vi "Teleop.vi"(0 "Call Context":T11, 1 "Input":T1) -> (6 "SubState 3":T5, 8 "SubState 4":T5, 9 "SubState 5":T10, 11 "Loop 3 Data":T6, 13 "Loop 4 Data":T4, 14 "SubState 0":T5=enum."driver control", 15 "Loop 1 Data":T8, 16 "Loop 0 Data":T9, 17 "SubState 1":T5, 18 "Loop 2 Data":T7, 19 "SubState 2":T5)   [LabVIEW 2013]
uses:
  typedefs/subStates.ctl
  <vilib>/Rock Robotics/WPI/DriverStation/WPI_DriverStationDerivedRobotMode.ctl
  typedefs/singleUseSubstate.ctl
  typedefs/Loop Datatypes/Loop 0 Datatype.ctl
  typedefs/Loop Datatypes/Loop 1 Datatype.ctl
  typedefs/Loop Datatypes/Loop 2 Datatype.ctl
  typedefs/Loop Datatypes/Loop 3 Datatype.ctl
  typedefs/Loop Datatypes/Loop 4 Datatype.ctl
  <vilib>/Rock Robotics/WPI/Joystick/WPI_JoystickDevRef.ctl
  <vilib>/Rock Robotics/WPI/Joystick/WPI_JoystickDeviceEnum.ctl
  <vilib>/Rock Robotics/WPI/Joystick/WPI_JoystickGetSetRefNum.vi
panel:
  out "JS Axis 2":dbl
  out "JS Axis 1":dbl
  out "JS3":T2
  out "JS1":T2
  out "JS2":T2
  out "Exit Value":i32=-1
  # "Loop Data and Substates"
  # "Latch Loop"
  # "Drive Loop"
  # "Shooter Pneumatics Loop"
  # "Pickup/Passing Belts Loop"
  # "Pickup Arm Loop"
  # "Shifter Loop"
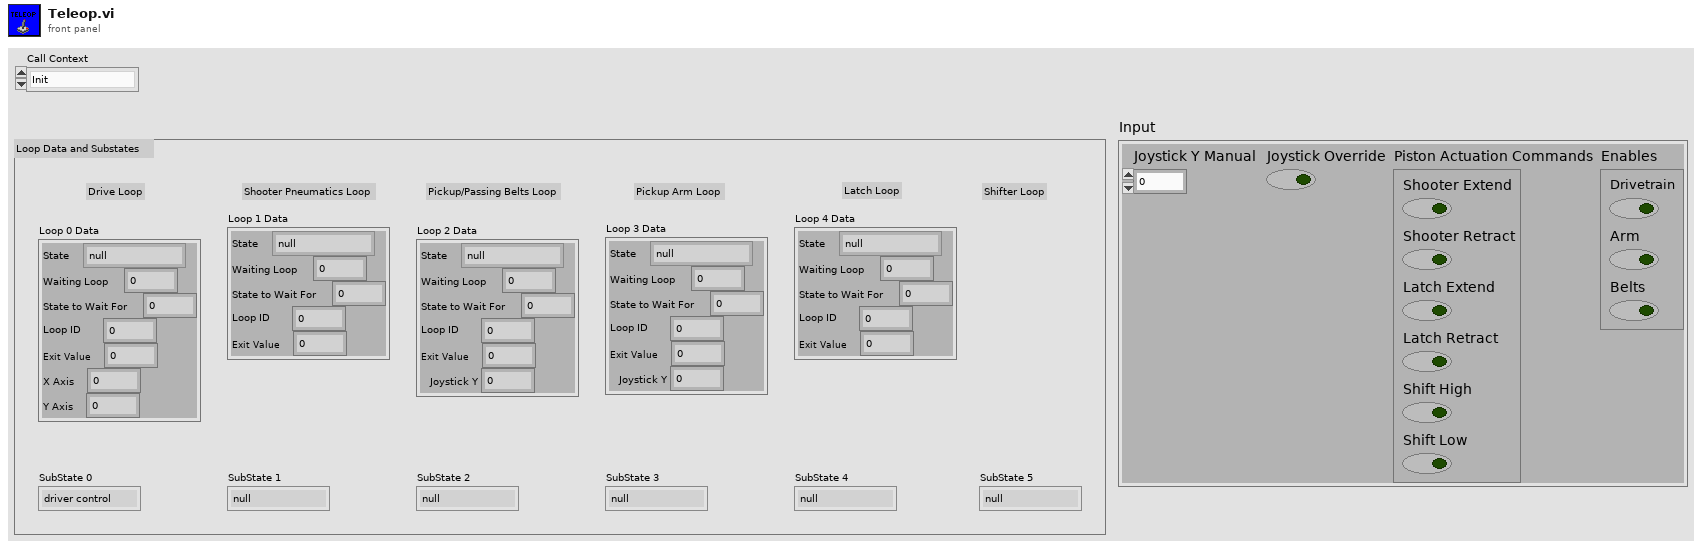
[diagram p1: front panel]
types:
  T1 = cluster{"Joystick Y Manual":dbl, "Joystick Override":bool, "Piston Actuation Commands":cluster{"Shooter Extend":bool, "Shooter Retract":bool, "Latch Extend":bool, "Latch Retract":bool, "Shift High":bool, "Shift Low":bool}, "Enables":cluster{"Drivetrain":bool, "Arm":bool, "Belts":bool}}
  T2 = typedef "WPI_JoystickDevRef.ctl" = cluster{"Device":T3}
  T3 = typedef "WPI_JoystickDeviceEnum.ctl" = enum16{"USB 1", "USB 2", "USB 3", "USB 4", "Kinect 1", "Kinect 2"}
  T4 = typedef "Loop 4 Datatype.ctl" = cluster{"State":T5, "Waiting Loop":i32, "State to Wait For":i32, "Loop ID":i32, "Exit Value":i32}
  T5 = typedef "subStates.ctl" = enum16{"null", "wait", "driver control", "auto", "manual override", "hold position", "rotate", "pickup", "pass", "load", "goto shoot", "shoot", "cancel", "end"}
  T6 = typedef "Loop 3 Datatype.ctl" = cluster{"State":T5, "Waiting Loop":i32, "State to Wait For":i32, "Loop ID":i32, "Exit Value":i32, "Joystick Y":dbl}
  T7 = typedef "Loop 2 Datatype.ctl" = cluster{"State":T5, "Waiting Loop":i32, "State to Wait For":i32, "Loop ID":i32, "Exit Value":i32, "Joystick Y":dbl}
  T8 = typedef "Loop 1 Datatype.ctl" = cluster{"State":T5, "Waiting Loop":i32, "State to Wait For":i32, "Loop ID":i32, "Exit Value":i32}
  T9 = typedef "Loop 0 Datatype.ctl" = cluster{"State":T5, "Waiting Loop":i32, "State to Wait For":i32, "Loop ID":i32, "Exit Value":i32, "X Axis":dbl, "Y Axis":dbl}
  T10 = typedef "singleUseSubstate.ctl" = enum16{"null", "wait", "shift high", "shift low"}
  T11 = typedef "WPI_DriverStationDerivedRobotMode.ctl" = enum16{"Init", "Execute", "Stop"}
  T12 = cluster{"Shooter Extend":bool, "Shooter Retract":bool, "Latch Extend":bool, "Latch Retract":bool, "Shift High":bool, "Shift Low":bool}
  T13 = cluster{"Drivetrain":bool, "Arm":bool, "Belts":bool}
  T14 = cluster{"axis 1 (x)":dbl, "axis 2 (y)":dbl, "axis 3 (throttle)":dbl, "axis 4":dbl, "axis 5":dbl, "axis 6":dbl}
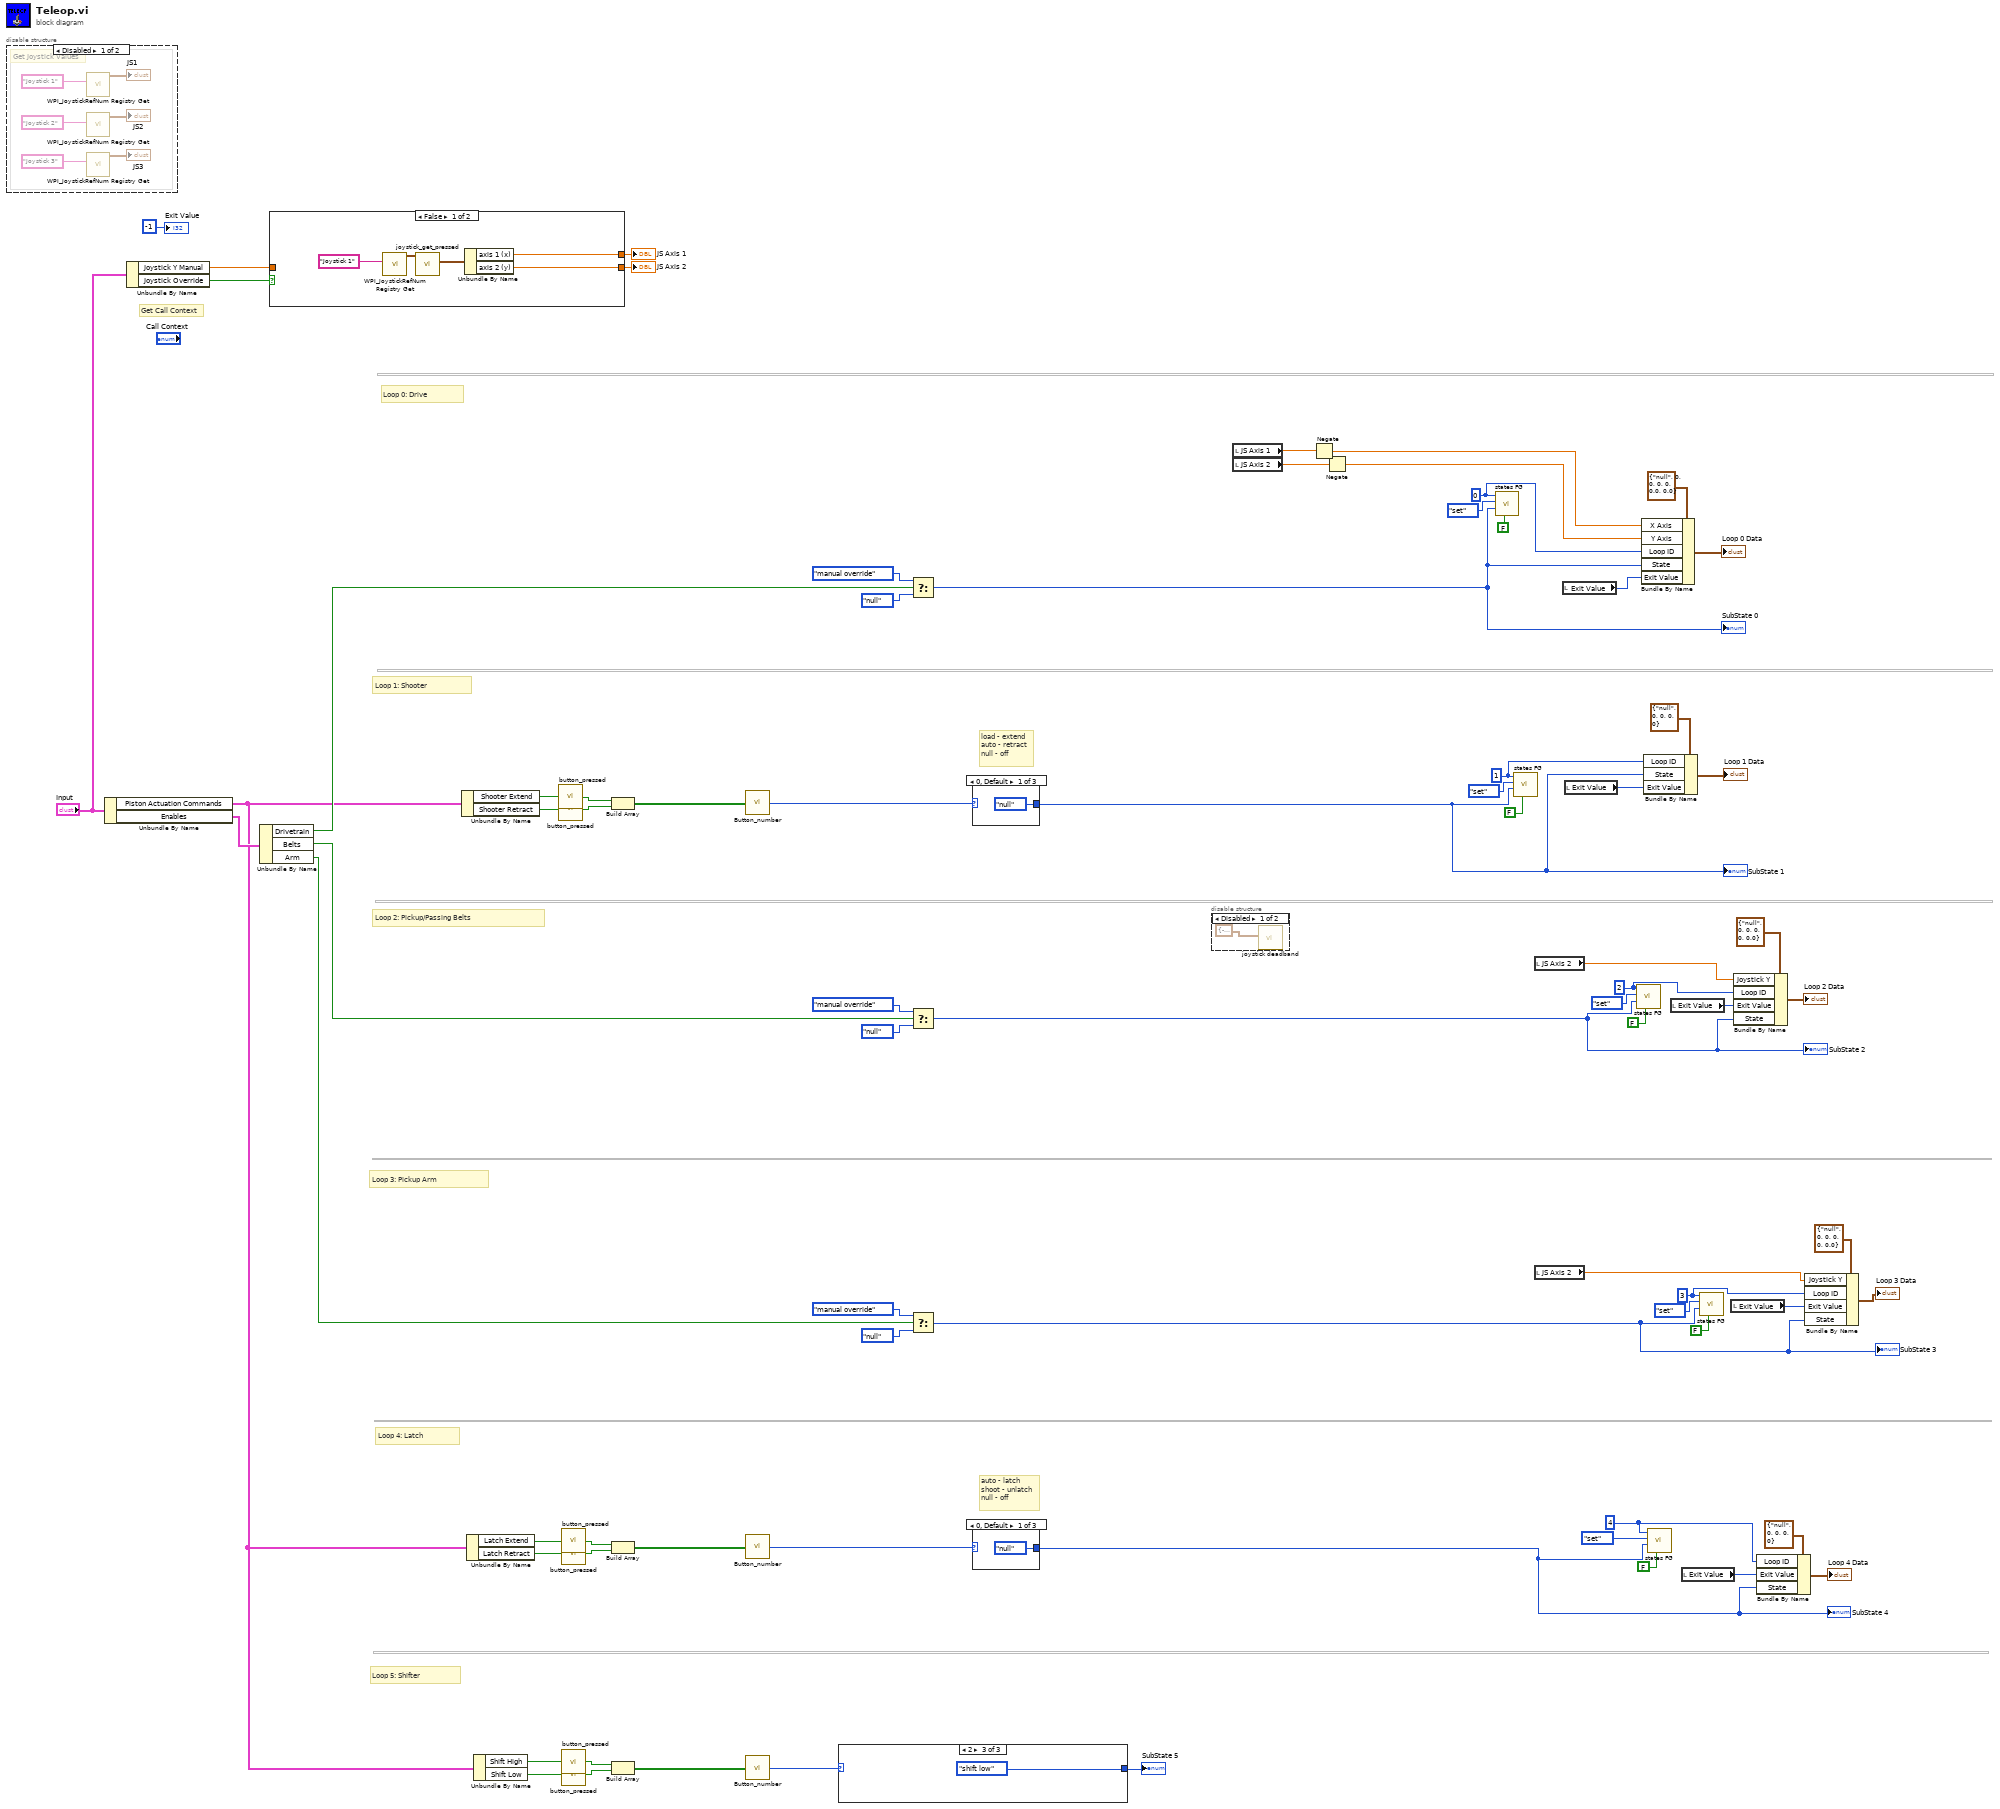
[diagram p0: block diagram]
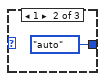
[diagram p5: hidden frame]
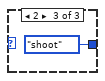
[diagram p6: hidden frame]
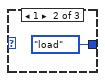
[diagram p7: hidden frame]
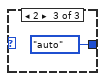
[diagram p8: hidden frame]
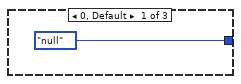
[diagram p9: hidden frame]
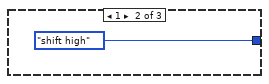
[diagram p10: hidden frame]
diagram:
  w45 = 4 ("Loop ID")
  w58 = 3 ("Loop ID")
  w59 = 2 ("Loop ID")
  w68 = 1 ("Loop ID")
  w70 = 0 ("Loop ID")
  # "auto - latch\nshoot - unlatch\nnull - off"
  # "load - extend\nauto - retract\nnull - off"
  # "Get Call Context"
  # "Loop 4: Latch"
  # "Loop 3: Pickup Arm"
  # "Loop 5: Shifter"
  # "Loop 2: Pickup/Passing Belts"
  # "Loop 1: Shooter"
  # "Loop 0: Drive"
  n1 = disable-structure shown="Disabled" {
    frame Disabled {
      # "Get Joystick Values"
      n2 = call <vilib>:"WPI_JoystickRefNum Registry Get.vi"("refnum name"="Joystick 1") -> ("JoystickDevRef"=→"JS1":T2)  [unwired: 9 in, 1 out]
      n3 = call <vilib>:"WPI_JoystickRefNum Registry Get.vi"("refnum name"="Joystick 2") -> ("JoystickDevRef"=→"JS2":T2)  [unwired: 9 in, 1 out]
      n4 = call <vilib>:"WPI_JoystickRefNum Registry Get.vi"("refnum name"="Joystick 3") -> ("JoystickDevRef"=→"JS3":T2)  [unwired: 9 in, 1 out]
    }
    frame Enabled {
    }
  }
  n5 = Unbundle By Name("Input") -> ("Piston Actuation Commands"=w22:T12, "Enables"=w43:T13)
  n6 = Unbundle By Name("Input") -> ("Joystick Y Manual"=w19:dbl, "Joystick Override"=w20:bool)
  n7 = Unbundle By Name(w43) -> ("Drivetrain"=w42:bool, "Belts"=w36:bool, "Arm"=w31:bool)
  n8 = case shown="False" w20 {
    tunnel: w19 -> [_ w89]
    tunnel: [w84 w89] -> w17
    tunnel: [w85 w89] -> w18
    frame False {
      n9 = call <vilib>:"WPI_JoystickRefNum Registry Get.vi"("refnum name"="Joystick 1") -> ("JoystickDevRef"=w87:T2)  [unwired: 9 in, 1 out]
      n10 = call "joystick_get_pressed.vi"("JoystickDevRef 2"=w87) -> ("Axes"=w86:T14)  [unwired: 1 in, 3 out]
      n11 = Unbundle By Name(w86) -> ("axis 1 (x)"=w85:dbl, "axis 2 (y)"=w84:dbl)
    }
    frame True {
    }
  }
  "JS Axis 1" <- w18
  "JS Axis 2" <- w17
  n12 = Unbundle By Name(w22) -> ("Shooter Extend"=w12:bool, "Shooter Retract"=w10:bool)
  n13 = Unbundle By Name(w22) -> ("Latch Extend"=w7:bool, "Latch Retract"=w8:bool)
  n14 = Unbundle By Name(w22) -> ("Shift High"=w3:bool, "Shift Low"=w4:bool)
  n15 = call "button_pressed.vi"("Button In"=w12) -> ("Button Pressed?"=w11:bool)
  n16 = call "button_pressed.vi"("Button In"=w10) -> ("Button Pressed?"=w9:bool)
  n17 = call "button_pressed.vi"("Button In"=w7) -> ("Button Pressed?"=w6:bool)
  n18 = call "button_pressed.vi"("Button In"=w8) -> ("Button Pressed?"=w5:bool)
  n19 = call "button_pressed.vi"("Button In"=w3) -> ("Button Pressed?"=w2:bool)
  n20 = call "button_pressed.vi"("Button In"=w4) -> ("Button Pressed?"=w1:bool)
  n21 = Build Array(w11, w9) -> (w30:bool[])
  n22 = Build Array(w6, w5) -> (w26:bool[])
  n23 = Build Array(w2, w1) -> (w24:bool[])
  n24 = call "Button_number.vi"("Button Array"=w30) -> ("Button Pressed"=w29:i32)
  n25 = call "Button_number.vi"("Button Array"=w26) -> ("Button Pressed"=w27:i32)
  n26 = call "Button_number.vi"("Button Array"=w24) -> ("Button Pressed"=w23:i32)
  n27 = case shown="2" w23 {
    tunnel: [singleUseSubstate."null" ("Enum") singleUseSubstate."shift high" ("Enum") singleUseSubstate."shift low" ("Enum")] -> w51
    frame 0, Default {
    }
    frame 1 {
    }
    frame 2 {
    }
  }
  "SubState 5" <- w51
  n28 = Select(t=subStates."manual override" ("Drive SubState"), s=w42, f=subStates."null" ("Drive SubState")) -> (s? t:f=w39:T5)
  "SubState 0" <- w39
  n29 = Select(t=subStates."manual override" ("Drive SubState"), s=w36, f=subStates."null" ("Drive SubState")) -> (s? t:f=w35:T5)
  "SubState 2" <- w35
  n30 = Select(t=subStates."manual override" ("Drive SubState"), s=w31, f=subStates."null" ("Drive SubState")) -> (s? t:f=w32:T5)
  "SubState 3" <- w32
  n31 = case shown="0, Default" w29 {
    tunnel: [subStates."null" ("Drive SubState") subStates."load" ("Drive SubState") subStates."auto" ("Drive SubState")] -> w28
    frame 0, Default {
    }
    frame 1 {
    }
    frame 2 {
    }
  }
  "SubState 1" <- w28
  n32 = case shown="0, Default" w27 {
    tunnel: [subStates."null" ("Drive SubState") subStates."auto" ("Drive SubState") subStates."shoot" ("Drive SubState")] -> w25
    frame 0, Default {
    }
    frame 1 {
    }
    frame 2 {
    }
  }
  "SubState 4" <- w25
  n33 = disable-structure shown="Disabled" {
    frame Disabled {
      n34 = call "joystick deadband.vi"("Deadband Range"=cluster{"Deadband Min":dbl, "Deadband Max":dbl} {"Deadband Min"=-0.05, "Deadband Max"=0.05}) -> ()  [unwired: 5 in, 1 out]
    }
    frame Enabled {
    }
  }
  n35 = local read "JS Axis 1"() -> (w16:dbl)
  n36 = local read "JS Axis 2"() -> (w15:dbl)
  n37 = Negate(x=w16) -> (-x=w50:dbl)
  n38 = Negate(x=w15) -> (-x=w49:dbl)
  n39 = call "states FG.vi"("exit in"=FALSE, "subState in"=w39, "menu (get)"=enum16{"set", "get"}."set", "Loop ID"=w70) -> ()  [unwired: 4 in, 4 out]
  n40 = call "states FG.vi"("exit in"=FALSE, "subState in"=w28, "menu (get)"=enum16{"set", "get"}."set", "Loop ID"=w68) -> ()  [unwired: 4 in, 4 out]
  n41 = local read "JS Axis 2"() -> (w14:dbl)
  n42 = local read "JS Axis 2"() -> (w13:dbl)
  n43 = local read "Exit Value"() -> (w66:i32)
  n44 = local read "Exit Value"() -> (w65:i32)
  n45 = call "states FG.vi"("exit in"=FALSE, "subState in"=w35, "menu (get)"=enum16{"set", "get"}."set", "Loop ID"=w59) -> ()  [unwired: 4 in, 4 out]
  n46 = Bundle By Name(cluster=T9 {"State"=enum."null", "Waiting Loop"=0, "State to Wait For"=0, "Loop ID"=0, "Exit Value"=0, "X Axis"=0.0, "Y Axis"=0.0} ("Cluster"), "X Axis"=w50, "Y Axis"=w49, "Loop ID"=w70, "State"=w39, "Exit Value"=w66) -> (→"Loop 0 Data":T9)
  n47 = Bundle By Name(cluster=T8 {"State"=enum."null", "Waiting Loop"=0, "State to Wait For"=0, "Loop ID"=0, "Exit Value"=0} ("Cluster"), "Loop ID"=w68, "State"=w28, "Exit Value"=w65) -> (→"Loop 1 Data":T8)
  n48 = call "states FG.vi"("exit in"=FALSE, "subState in"=w25, "menu (get)"=enum16{"set", "get"}."set", "Loop ID"=w45) -> ()  [unwired: 4 in, 4 out]
  n49 = local read "Exit Value"() -> (w60:i32)
  n50 = local read "Exit Value"() -> (w46:i32)
  n51 = call "states FG.vi"("exit in"=FALSE, "subState in"=w32, "menu (get)"=enum16{"set", "get"}."set", "Loop ID"=w58) -> ()  [unwired: 4 in, 4 out]
  n52 = local read "Exit Value"() -> (w57:i32)
  n53 = Bundle By Name(cluster=T7 {"State"=enum."null", "Waiting Loop"=0, "State to Wait For"=0, "Loop ID"=0, "Exit Value"=0, "Joystick Y"=0.0} ("Loop 2 Data"), "Joystick Y"=w14, "Loop ID"=w59, "Exit Value"=w60, "State"=w35) -> (→"Loop 2 Data":T7)
  n54 = Bundle By Name(cluster=T4 {"State"=enum."null", "Waiting Loop"=0, "State to Wait For"=0, "Loop ID"=0, "Exit Value"=0} ("Loop 4 Data"), "Loop ID"=w45, "Exit Value"=w46, "State"=w25) -> (→"Loop 4 Data":T4)
  n55 = Bundle By Name(cluster=T6 {"State"=enum."null", "Waiting Loop"=0, "State to Wait For"=0, "Loop ID"=0, "Exit Value"=0, "Joystick Y"=0.0} ("Loop 3 Data"), "Joystick Y"=w13, "Loop ID"=w58, "Exit Value"=w57, "State"=w32) -> (→"Loop 3 Data":T6)
  "Exit Value" <- -1 ("Exit Value")
